vi "ROS_Subscribers.vi"() -> ()   [LabVIEW 2016]
doc: "The ROS Subscriber subscribes to two topics, the unicorn current state and the intention variable from the local planner."
uses:
  <userlib>/ROS for LabVIEW Software/ROS/Code/Console/Servers/ServerSubs/TopicDef.ctl
  <userlib>/ROS for LabVIEW Software/ROS/Code/SubVIs/_ROSDirection.ctl
  GlobalVI.vi
  <userlib>/ROS for LabVIEW Software/ROS/MessageParsing/std_msgs/subs/parse_i32_scalar.vi
  <userlib>/ROS for LabVIEW Software/ROS/Code/_ROSDefinition.vi
panel:
  out "\\TX2_unicorn_state":i32
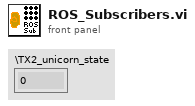
[diagram p1: front panel]
types:
  T1 = typedef "TopicDef.ctl" = cluster{"Topic":string, "Type":string, "Action":T2, "Update (ms)":u16, "queue size":u16}
  T2 = typedef "_ROSDirection.ctl" = enum16{"Node", "Publisher", "Subscriber", "ServiceClient", "ServiceProvider"}
  T3 = typedef "_ROSControl.ctl" = cluster{"topic port":u16, "Node":string, "topic":string, "type":string, "node port":u16, "error ":errorcluster, "Direction":T2, "Update (ms)":u16, "FIFO size":u16}
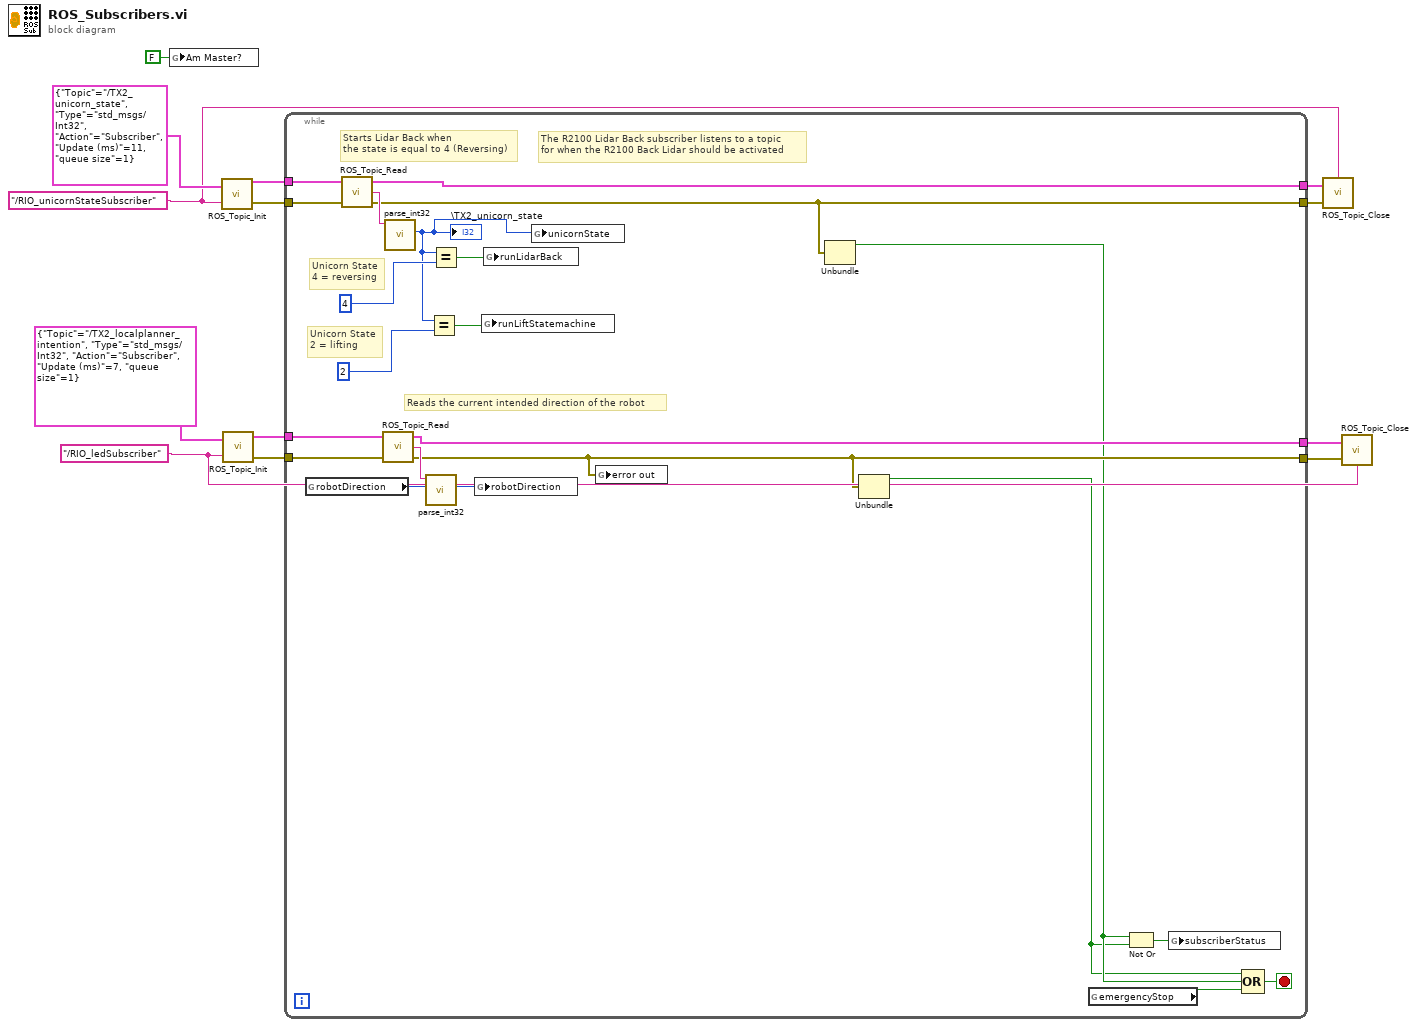
[diagram p0: block diagram]
diagram:
  w7 = "/RIO_ledSubscriber" ("node")
  w9 = "/RIO_unicornStateSubscriber" ("node")
  n1 = global write "_ROSDefinition.vi" "Am Master?"(FALSE ("Am Master?")) -> ()
  n2 = call <userlib>:"ROS_Topic_Init.vi"("Definitions"=T1 {"Topic"="/TX2_unicorn_state", "Type"="std_msgs/Int32", "Action"=enum."Subscriber", "Update (ms)"=11, "queue size"=1}, "node"=w9) -> ("ROS out"=w12:T3, "error out"=w1:errorcluster)  [unwired: 1 in]
  n3 = call <userlib>:"ROS_Topic_Init.vi"("Definitions"=T1 {"Topic"="/TX2_localplanner_intention", "Type"="std_msgs/Int32", "Action"=enum."Subscriber", "Update (ms)"=7, "queue size"=1}, "node"=w7) -> ("ROS out"=w6:T3, "error out"=w2:errorcluster)  [unwired: 1 in]
  n4 = while {
    tunnel: w12 -> [w35]
    tunnel: [w33] -> w10
    tunnel: w1 -> [w34]
    tunnel: [w20] -> w11
    tunnel: w6 -> [w25]
    tunnel: w2 -> [w24]
    tunnel: [w19] -> w5
    tunnel: [w23] -> w4
    stop <- w18 stop-if-true
    # "The R2100 Lidar Back subscriber listens to a topic \nfor when the R2100 Back Lidar should be activated"
    # "Reads the current intended direction of the robot"
    # "Unicorn State\n2 = lifting"
    # "Unicorn State\n4 = reversing"
    # "Starts Lidar Back when\nthe state is equal to 4 (Reversing)"
    n5 = global read "GlobalVI.vi" "robotDirection"() -> (w21:i32)
    n6 = call <userlib>:"ROS_Topic_Read.vi"("error in (no error)"=w34, "ROS in"=w35) -> ("error out"=w20:errorcluster, "Reply"=w32:string, "ROS out"=w33:T3)  [unwired: 1 in]
    n7 = call <userlib>:"ROS_Topic_Read.vi"("error in (no error)"=w24, "ROS in"=w25) -> ("error out"=w19:errorcluster, "Reply"=w26:string, "ROS out"=w23:T3)  [unwired: 1 in]
    n8 = call-poly <userlib>:"parse_int32.vi"("msg in"=w32) -> ("number"=w27:i32)  [unwired: 4 in, 2 out]
    "\\TX2_unicorn_state" <- w27
    n9 = call-poly <userlib>:"parse_int32.vi"("type"=w21, "msg in"=w26) -> ("number"=w22:i32)  [unwired: 3 in, 2 out]
    n10 = Equal?(x=w27, y=2) -> (x = y?=w28:bool)
    n11 = Equal?(x=w27, y=4) -> (x = y?=w30:bool)
    n12 = global write "GlobalVI.vi" "robotDirection"(w22) -> ()
    n13 = global write "GlobalVI.vi" "runLiftStatemachine"(w28) -> ()
    n14 = global write "GlobalVI.vi" "runLidarBack"(w30) -> ()
    n15 = global write "GlobalVI.vi" "unicornState"(w27) -> ()
    n16 = global write "GlobalVI.vi" "error out"(w19) -> ()
    n17 = Unbundle(w20) -> ("status"=w16:bool)  [unwired: 2 out]
    n18 = Unbundle(w19) -> ("status"=w15:bool)  [unwired: 2 out]
    n19 = global read "GlobalVI.vi" "emergencyStop"() -> (w17:bool)
    n20 = Not Or(1:w15, 2:w16) -> (0:w14:bool)
    n21 = global write "GlobalVI.vi" "subscriberStatus"(w14) -> ()
    n22 = Compound Arithmetic op=OR(w15, w16, w17) -> (w18:bool)
  }
  n23 = call <userlib>:"ROS_Topic_Close.vi"("error in"=w11, "ROS in"=w10, "node"=w9) -> ()  [unwired: 1 in, 1 out]
  n24 = call <userlib>:"ROS_Topic_Close.vi"("error in"=w5, "ROS in"=w4, "node"=w7) -> ()  [unwired: 1 in, 1 out]
